vi "Convert File Extension (Path).vi"(2 "new ending (none)":string, 3 "file name":path) -> (0 "prev ending":string, 1 "new filename":path)   [LabVIEW 2015]
doc: "Converts the file extension of a file. \"new ending\" will accept an extension prefixed with or without a period, or a blank (\"\") string.\nFor example:\n\nfile name => c:\\temp\\data.txt\nnew ending => \"csv\" or \".csv\"\nnew filename => c:\\temp\\data.csv\nprev ending => \".txt\"\n\nfile name => c:\\temp\\data.txt\nnew ending => \"\"\nnew filename => c:\\temp\\data\nprev ending => \".txt\""
panel:
  # "Convert File Extension.vi\n\nConverts the file extension of a file\n\nPlease visit http://www.OpenG.org to learn about the\nOpen Source LabVIEW software movement.\n\nNOTICE -- YOU MUST LEAVE THIS NOTICE IN PLACE.  PER THE TERMS OF THE LICENSE BELOW, YOU MAY SUBLICENSE THIS SOFTWARE \nIN ANY WAY THAT DOES NOT CONFLICT WITH THIS LICENSE.\n\n### BSD License (http://www.opensource.org/licenses/bsd-license.php) Begin ###\n\nCopyright (c) 2002, Rolf Kalbermatter <rolf.kalbermatter@citeng.com> \nCopyright (c) 2002-2006, Jim Kring <jim@jimkring.com>\n\nAll rights reserved.\n\nRedistribution and use in source and binary forms, with or without modification, are permitted provided that the following conditions are met:\n\n    * Redistributions of source code must retain the above copyright notice, this list of conditions and the following disclaimer.\n    * Redistributions in binary form must reproduce the above copyright notice, this list of conditions and the following disclaimer in the \n       documentation and/or other materials provided with the distribution.\n    * Neither the name of SciWare, James Kring, Inc., nor the names of its contributors may be used to endorse or promote products derived \n       from this software without specific prior written permission.\n\nTHIS SOFTWARE IS PROVIDED BY THE COPYRIGHT HOLDERS AND CONTRIBUTORS \"AS IS\" AND ANY EXPRESS OR IMPLIED WARRANTIES, \nINCLUDING, BUT NOT LIMITED TO, THE IMPLIED WARRANTIES OF MERCHANTABILITY AND FITNESS FOR A PARTICULAR PURPOSE ARE \nDISCLAIMED. IN NO EVENT SHALL THE COPYRIGHT OWNER OR CONTRIBUTORS BE LIABLE FOR ANY DIRECT, INDIRECT, INCIDENTAL,\n SPECIAL, EXEMPLARY, OR CONSEQUENTIAL DAMAGES (INCLUDING, BUT NOT LIMITED TO, PROCUREMENT OF SUBSTITUTE GOODS OR \nSERVICES; LOSS OF USE, DATA, OR PROFITS; OR BUSINESS INTERRUPTION) HOWEVER CAUSED AND ON ANY THEORY OF LIABILITY, \nWHETHER IN CONTRACT, STRICT LIABILITY, OR TORT (INCLUDING NEGLIGENCE OR OTHERWISE) ARISING IN ANY WAY OUT OF THE USE \nOF THIS SOFTWARE, EVEN IF ADVISED OF THE POSSIBILITY OF SUCH DAMAGE.\n\n### BSD License End ###"
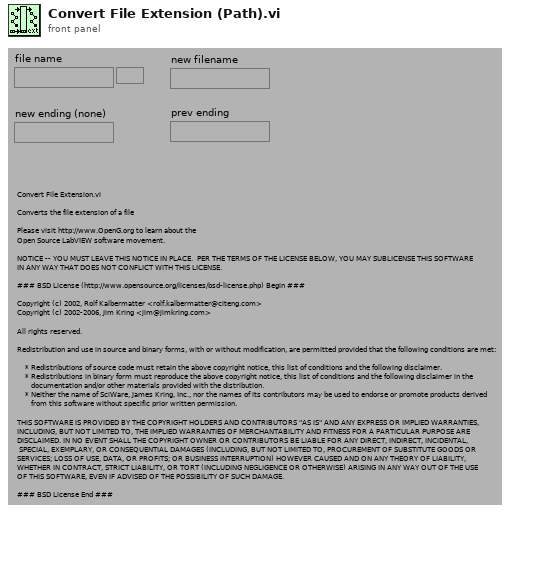
[diagram p1: front panel]
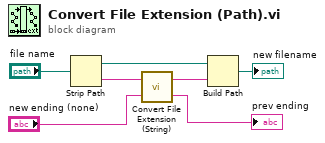
[diagram p0: block diagram]
diagram:
  n1 = Strip Path(path="file name") -> (stripped path=w3:path, name=w6:string)
  n2 = call "Convert File Extension (String).vi"("new ending (none)"="new ending (none)", "file name"=w6) -> ("prev ending"=→"prev ending":string, "new filename"=w4:string)
  n3 = Build Path(base path=w3, name or relative path=w4) -> (appended path=→"new filename":path)
